vi "LUCS001RT_GPS_Decoder_GPGLL.vi"(8 "error in (no error)":errorcluster, 9 "SerialData: GPGLL":string=",3751.65,S,14507.36,E*77", 11 "GPS Data In":T1={"WayPointDataGood"=TRUE, "Waypoint:XTE"=0.01, "Waypoint:SteeringDirection"="L", "WayPoint:OriginID"="", "Waypoint:DestinationID"="", "DestinationWaypoint.Latitude.Deg"=0, "DestinationWaypoint.Latitude.Min"=0.0, "DestinationWaypointLatitude.North/South"="", "DestinationWaypointLongitude.Deg"=0, "DestinationWaypointLongitude.Min"=0.0, "DestinationWaypointLongitude.East/West"="", "RangeToDestination(NauticalMiles)"=0.0, "TrueBearingToDestination"=33.7, "VelocityTowardsDestination(Knots)"=0.0, "ArrivalAlarm"=TRUE, "ITOW"=247, "TAcc"=0, "LON"=0.0, "LAT"=0.0, "HEIGHT"=0, "HMSL"=0, "Hacc"=0, "Vacc"=0, "MSTOW"=0, "FixType"=0, "ECEF_X_Coor"=0, "ECEF_Y_Coor"=0, "ECEF_Z_Coor"=0, "Pacc"=0, "ECEF_X_Vlsty"=0, "ECEF_Y_Vlsty"=0, "ECEF_Z_Vlsty"=0, "Sacc"=0, "PosDOP"=0, "#SatsInNavSol"=0, "NED_NVsty"=0, "NED_Evsty"=0, "NED_DNvsty"=0, "Speed(3-D)"=0, "GSpeed(2-D)"=0, "Heading(2-D)"=0.0, "CAcc"=0, "Nano"=0, "Year"=0, "Month"=0, "Day"=0, "Hour"=0, "Min"=0, "Sec"=0, "UTC Valid"=0} {"UTC Valid" items=["UTC not valid", "Valid Time of Week", "Valid Week Number", "NA", "Valid UTC"]; "CAcc" format="%.0f°"; "Heading(2-D)" format="%0.6f°"; "GSpeed(2-D)" format="%.0f cm/s"; "Speed(3-D)" format="%.0f cm/s"; "NED_DNvsty" format="%.0f cm/s"; "NED_Evsty" format="%.0f cm/s"; "NED_NVsty" format="%.0f cm/s"; "Sacc" format="%.0f cm/s"; "ECEF_Z_Vlsty" format="%.0f cm/s"; "ECEF_Y_Vlsty" format="%.0f cm/s"; "ECEF_X_Vlsty" format="%.0f cm/s"; "FixType" items=["No Fix", "Dead Reckoning Only", "2D-Fix", "3D-Fix", "GPS + Dead Reckoning", "Time Only Fix", "RESERVED"]; "Vacc" format="%.0f mm"; "Hacc" format="%.0f mm"; "HMSL" format="%d mm"; "HEIGHT" format="%.0f mm"; "LAT" format="%#.6f"; "LON" format="%#.6f"; "Waypoint:XTE" format="%#.2f"}) -> (0 "error out":errorcluster, 3 "GPS Data Out":T1={"WayPointDataGood"=TRUE, "Waypoint:XTE"=0.01, "Waypoint:SteeringDirection"="L", "WayPoint:OriginID"="", "Waypoint:DestinationID"="", "DestinationWaypoint.Latitude.Deg"=0, "DestinationWaypoint.Latitude.Min"=0.0, "DestinationWaypointLatitude.North/South"="", "DestinationWaypointLongitude.Deg"=0, "DestinationWaypointLongitude.Min"=0.0, "DestinationWaypointLongitude.East/West"="", "RangeToDestination(NauticalMiles)"=0.0, "TrueBearingToDestination"=33.7, "VelocityTowardsDestination(Knots)"=0.0, "ArrivalAlarm"=TRUE, "ITOW"=247, "TAcc"=0, "LON"=0.0, "LAT"=16.0, "HEIGHT"=0, "HMSL"=0, "Hacc"=0, "Vacc"=0, "MSTOW"=0, "FixType"=0, "ECEF_X_Coor"=0, "ECEF_Y_Coor"=0, "ECEF_Z_Coor"=0, "Pacc"=0, "ECEF_X_Vlsty"=0, "ECEF_Y_Vlsty"=0, "ECEF_Z_Vlsty"=0, "Sacc"=0, "PosDOP"=0, "#SatsInNavSol"=0, "NED_NVsty"=0, "NED_Evsty"=0, "NED_DNvsty"=0, "Speed(3-D)"=0, "GSpeed(2-D)"=0, "Heading(2-D)"=0.0, "CAcc"=0, "Nano"=0, "Year"=0, "Month"=0, "Day"=0, "Hour"=0, "Min"=0, "Sec"=0, "UTC Valid"=0} {"UTC Valid" items=["UTC not valid", "Valid Time of Week", "Valid Week Number", "NA", "Valid UTC"]; "CAcc" format="%.0f°"; "Heading(2-D)" format="%0.6f°"; "GSpeed(2-D)" format="%.0f cm/s"; "Speed(3-D)" format="%.0f cm/s"; "NED_DNvsty" format="%.0f cm/s"; "NED_Evsty" format="%.0f cm/s"; "NED_NVsty" format="%.0f cm/s"; "Sacc" format="%.0f cm/s"; "ECEF_Z_Vlsty" format="%.0f cm/s"; "ECEF_Y_Vlsty" format="%.0f cm/s"; "ECEF_X_Vlsty" format="%.0f cm/s"; "FixType" items=["No Fix", "Dead Reckoning Only", "2D-Fix", "3D-Fix", "GPS + Dead Reckoning", "Time Only Fix", "RESERVED"]; "Vacc" format="%.0f mm"; "Hacc" format="%.0f mm"; "HMSL" format="%d mm"; "HEIGHT" format="%.0f mm"; "LAT" format="%#.6f"; "LON" format="%#.6f"; "Waypoint:XTE" format="%#.2f"})   [LabVIEW 2020]
uses:
  LUCS001RT_GPS_Data.ctl
panel:
  # "WAYPOINT"
  # "CURRENT POSITION"
  # "WAYPOINT"
  # "CURRENT POSITION"
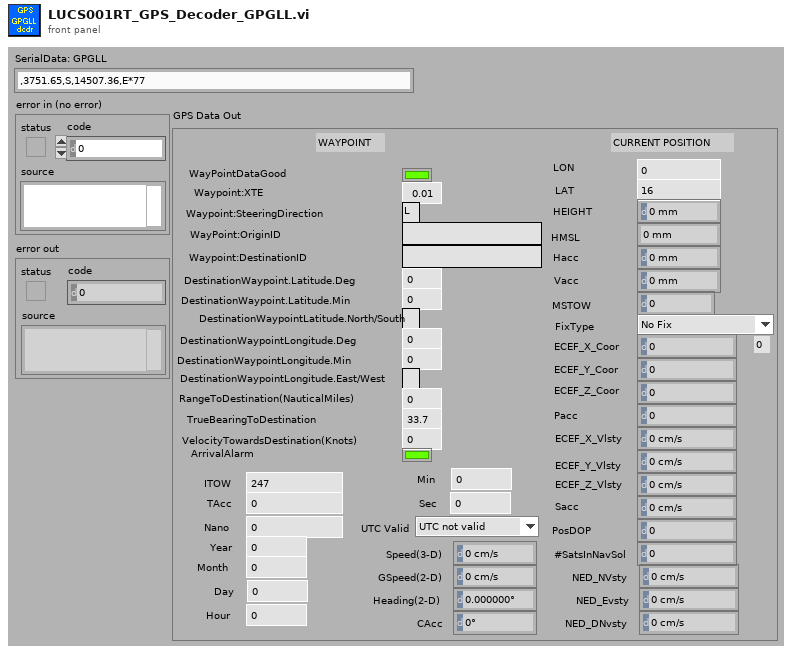
[diagram p1: front panel]
types:
  T1 = typedef "LUCS001RT_GPS_Data.ctl" = cluster{"WayPointDataGood":bool, "Waypoint:XTE":dbl, "Waypoint:SteeringDirection":string, "WayPoint:OriginID":string, "Waypoint:DestinationID":string, "DestinationWaypoint.Latitude.Deg":i32, "DestinationWaypoint.Latitude.Min":dbl, "DestinationWaypointLatitude.North/South":string, "DestinationWaypointLongitude.Deg":i32, "DestinationWaypointLongitude.Min":dbl, "DestinationWaypointLongitude.East/West":string, "RangeToDestination(NauticalMiles)":dbl, "TrueBearingToDestination":dbl, "VelocityTowardsDestination(Knots)":dbl, "ArrivalAlarm":bool, "ITOW":u32, "TAcc":u32, "LON":dbl, "LAT":dbl, "HEIGHT":i32, "HMSL":i32, "Hacc":u32, "Vacc":u32, "MSTOW":u32, "FixType":u8, "ECEF_X_Coor":i32, "ECEF_Y_Coor":i32, "ECEF_Z_Coor":i32, "Pacc":u32, "ECEF_X_Vlsty":i32, "ECEF_Y_Vlsty":i32, "ECEF_Z_Vlsty":i32, "Sacc":u32, "PosDOP":u16, "#SatsInNavSol":u8, "NED_NVsty":i32, "NED_Evsty":i32, "NED_DNvsty":i32, "Speed(3-D)":u32, "GSpeed(2-D)":u32, "Heading(2-D)":dbl, "CAcc":u32, "Nano":i32, "Year":u16, "Month":u8, "Day":u8, "Hour":u8, "Min":u8, "Sec":u8, "UTC Valid":u8}
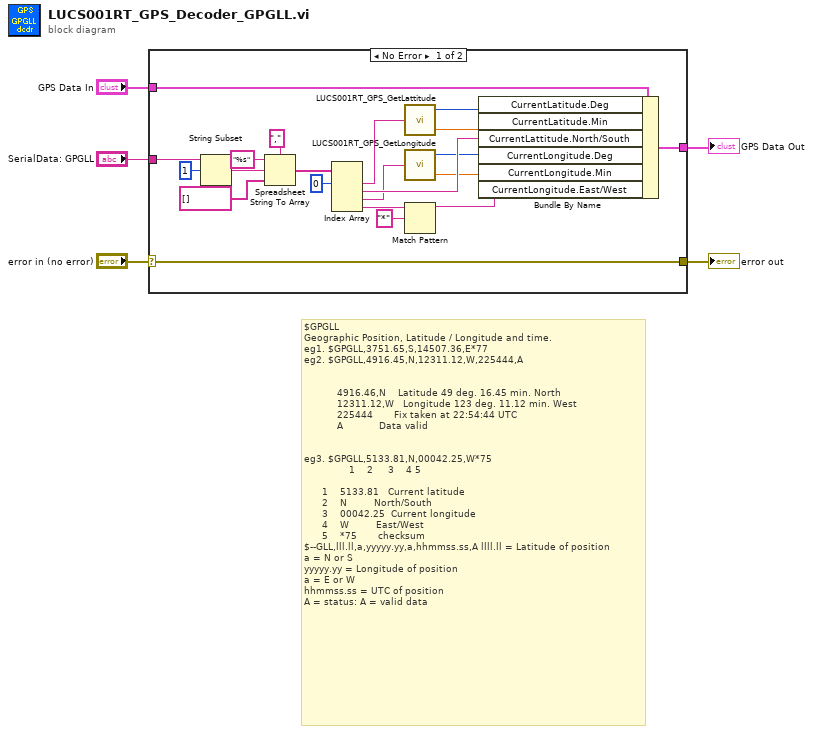
[diagram p0: block diagram]
diagram:
  # "$GPGLL\nGeographic Position, Latitude / Longitude and time. \neg1. $GPGLL,3751.65,S,14507.36,E*77\neg2. $GPGLL,4916.45,N,12311.12,W,225444,A\n\n\n           4916.46,N    Latitude 49 deg. 16.45 min. North\n           12311.12,W   Longitude 123 deg. 11.12 min. West\n           225444       Fix taken at 22:54:44 UTC\n           A            Data valid\n\n\neg3. $GPGLL,5133.81,N,00042.25,W*75\n               1    2     3    4 5\n\n      1    5133.81   Current latitude\n      2    N         North/South\n      3    00042.25  Current longitude\n      4    W         East/West\n      5    *75       checksum\n$--GLL,lll.ll,a,yyyyy.yy,a,hhmmss.ss,A llll.ll = Latitude of position \na = N or S \nyyyyy.yy = Longitude of position \na = E or W \nhhmmss.ss = UTC of position \nA = status: A = valid data"
  n1 = case shown="No Error" "error in (no error)" {
    selector: "error in (no error)" -> [w12 w27]
    tunnel: "SerialData: GPGLL" -> [w25 _]
    tunnel: "GPS Data In" -> [w16 _]
    tunnel: [w15 _] -> w3
    tunnel: [w12 w27] -> w1
    frame No Error {
      n2 = String Subset(string=w25, offset (0)=1) -> (substring=w21:string)  [unwired: 1 in]
      n3 = Spreadsheet String To Array(delimiter (Tab)=",", format string="%s", spreadsheet string=w21, array type (2D Dbl)=string[] []) -> (array=w26:string[])
      n4 = Index Array(array=w26, index #1=0 ("index")) -> (element #1=w11:string, element #2=w14:string, element #3=w8:string, element #4=w18:string)  [unwired: 3 in]
      n5 = call "LUCS001RT_GPS_GetLattitude.vi"("LattitudeString"=w11) -> ("Lattitude.Degrees"=w10:i32, "Lattitude.Minutes"=w9:dbl)  [unwired: 5 in]
      n6 = call "LUCS001RT_GPS_GetLongitude.vi"("LongitudeString"=w8) -> ("Longitude.Degrees"=w7:i32, "Longitude.Minutes"=w6:dbl)  [unwired: 5 in]
      n7 = Match Pattern(string=w18, regular expression="*") -> (before substring=w13:string)  [unwired: 1 in, 3 out]
      n8 = Bundle By Name(cluster=w16, "CurrentLatitude.Deg"=w10, "CurrentLatitude.Min"=w9, "CurrentLattitude.North/South"=w14, "CurrentLongitude.Deg"=w7, "CurrentLongitude.Min"=w6, "CurrentLongitude.East/West"=w13) -> (w15:T1)
    }
    frame Error {
    }
  }
  "GPS Data Out" <- w3
  "error out" <- w1
